vi "正式LABVIEW_11_16_1.vi"() -> ()   [LabVIEW 2019]
uses:
  <vilib>/Instr/_visa.llb/VISA Configure Serial Port (Instr).vi
panel:
  out "?":picture
  out "?":picture
  in  "防撞":bool
  out "右前":dbl
  out "左前":dbl
  out "オ":dbl
  out "右":dbl
  in  "更新影片&影片重播":bool
  in  "選擇導覽目標":path
  in  "導覽影片":refnum<k7>(container)
  out "濕度值":string
  in  "輸入阜來源":refnum<visa-resource-name>
  in  "指紋辨識成功影片":refnum<k7>(container)
  in  "指紋辨識檔案":path
  out "溫度值":string
  out "濕度條":dbl(slide) scale=0.0..100.0
  out "溫度條":dbl(slide) scale=0.0..50.0
  out "右後":dbl
  out "左後":dbl
  in  "倒車雷達":bool
  in  "溫度濕度開關":bool
  in  "程式關閉":bool
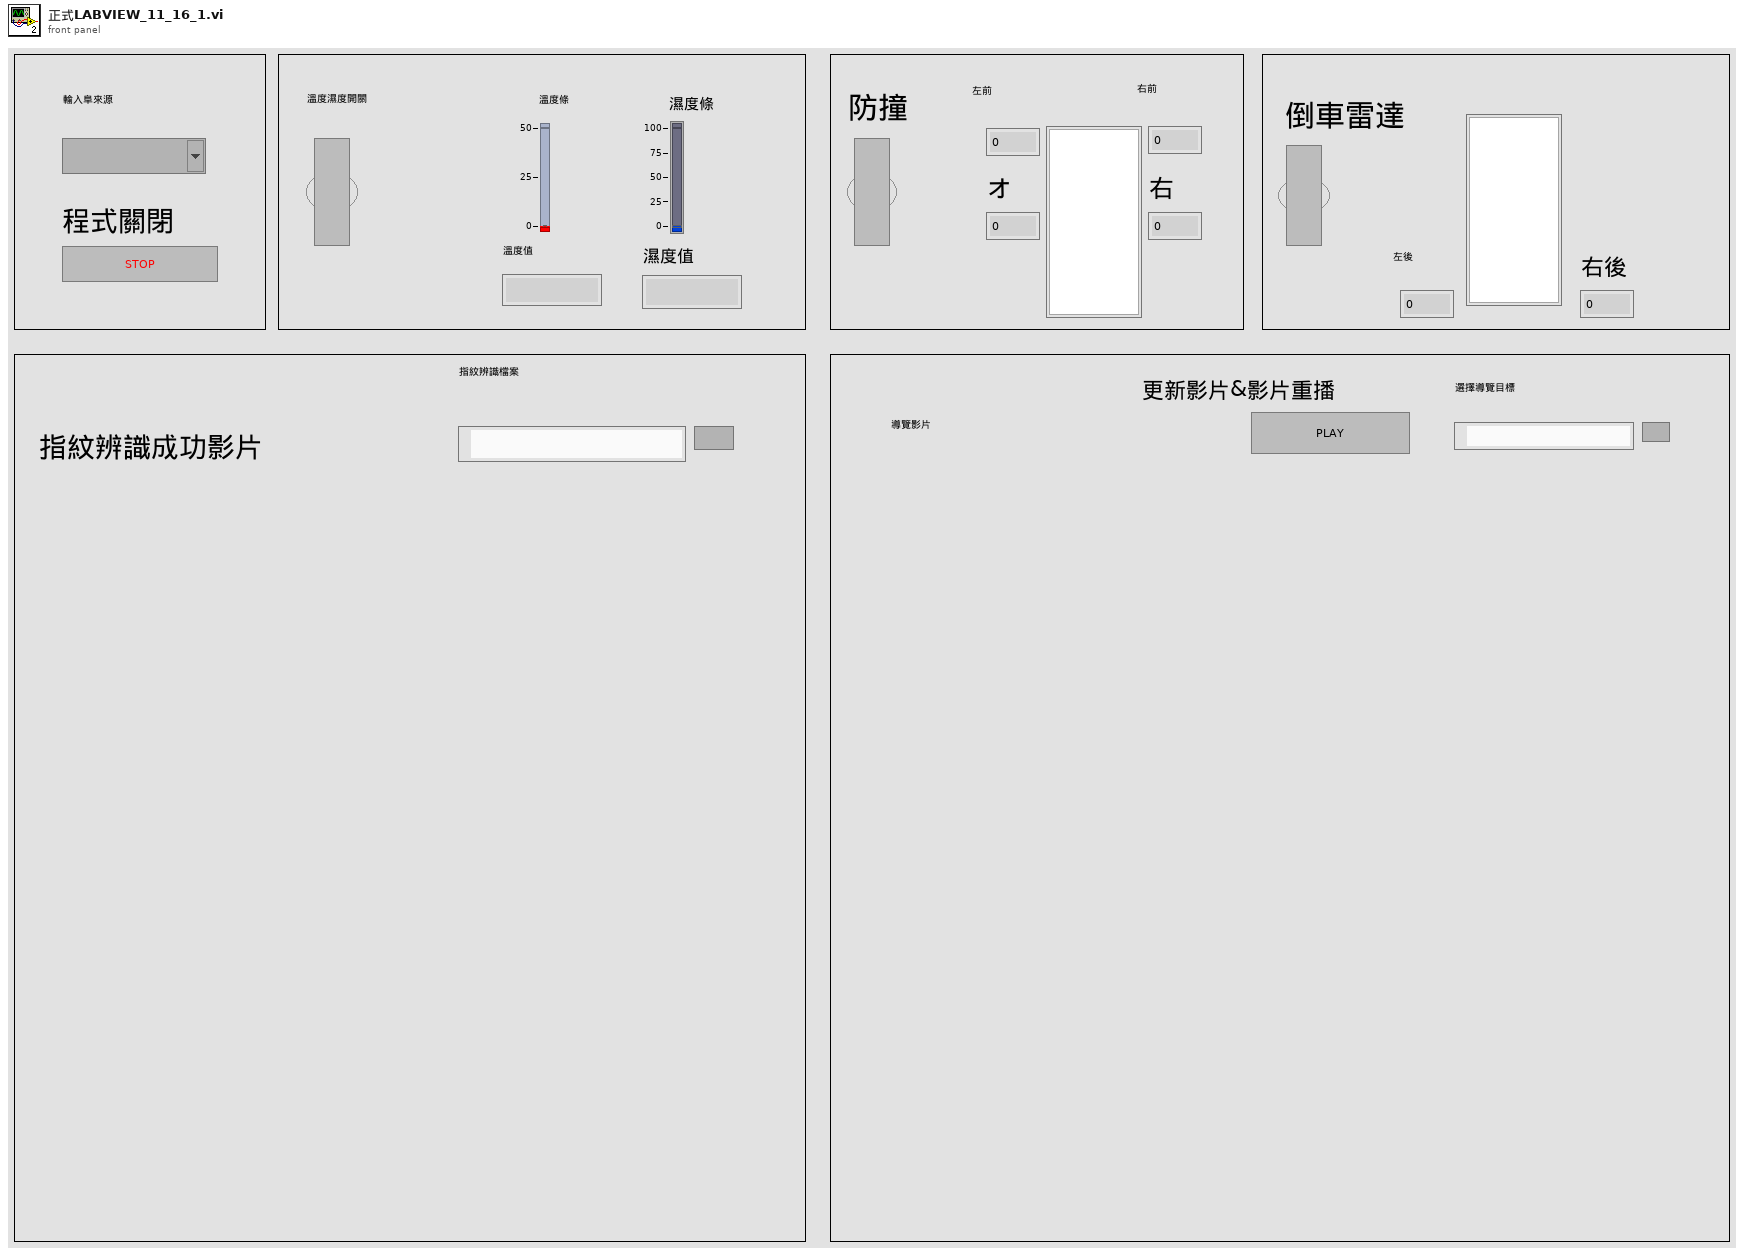
[diagram p1: front panel]
types:
  T1 = typedef "imagedata.ctl" = cluster{"image type":i32, "image depth":i32, "image":u8[], "mask":u8[], "colors":u32[], "Rectangle":cluster{"left":i16, "top":i16, "right":i16, "bottom":i16}}
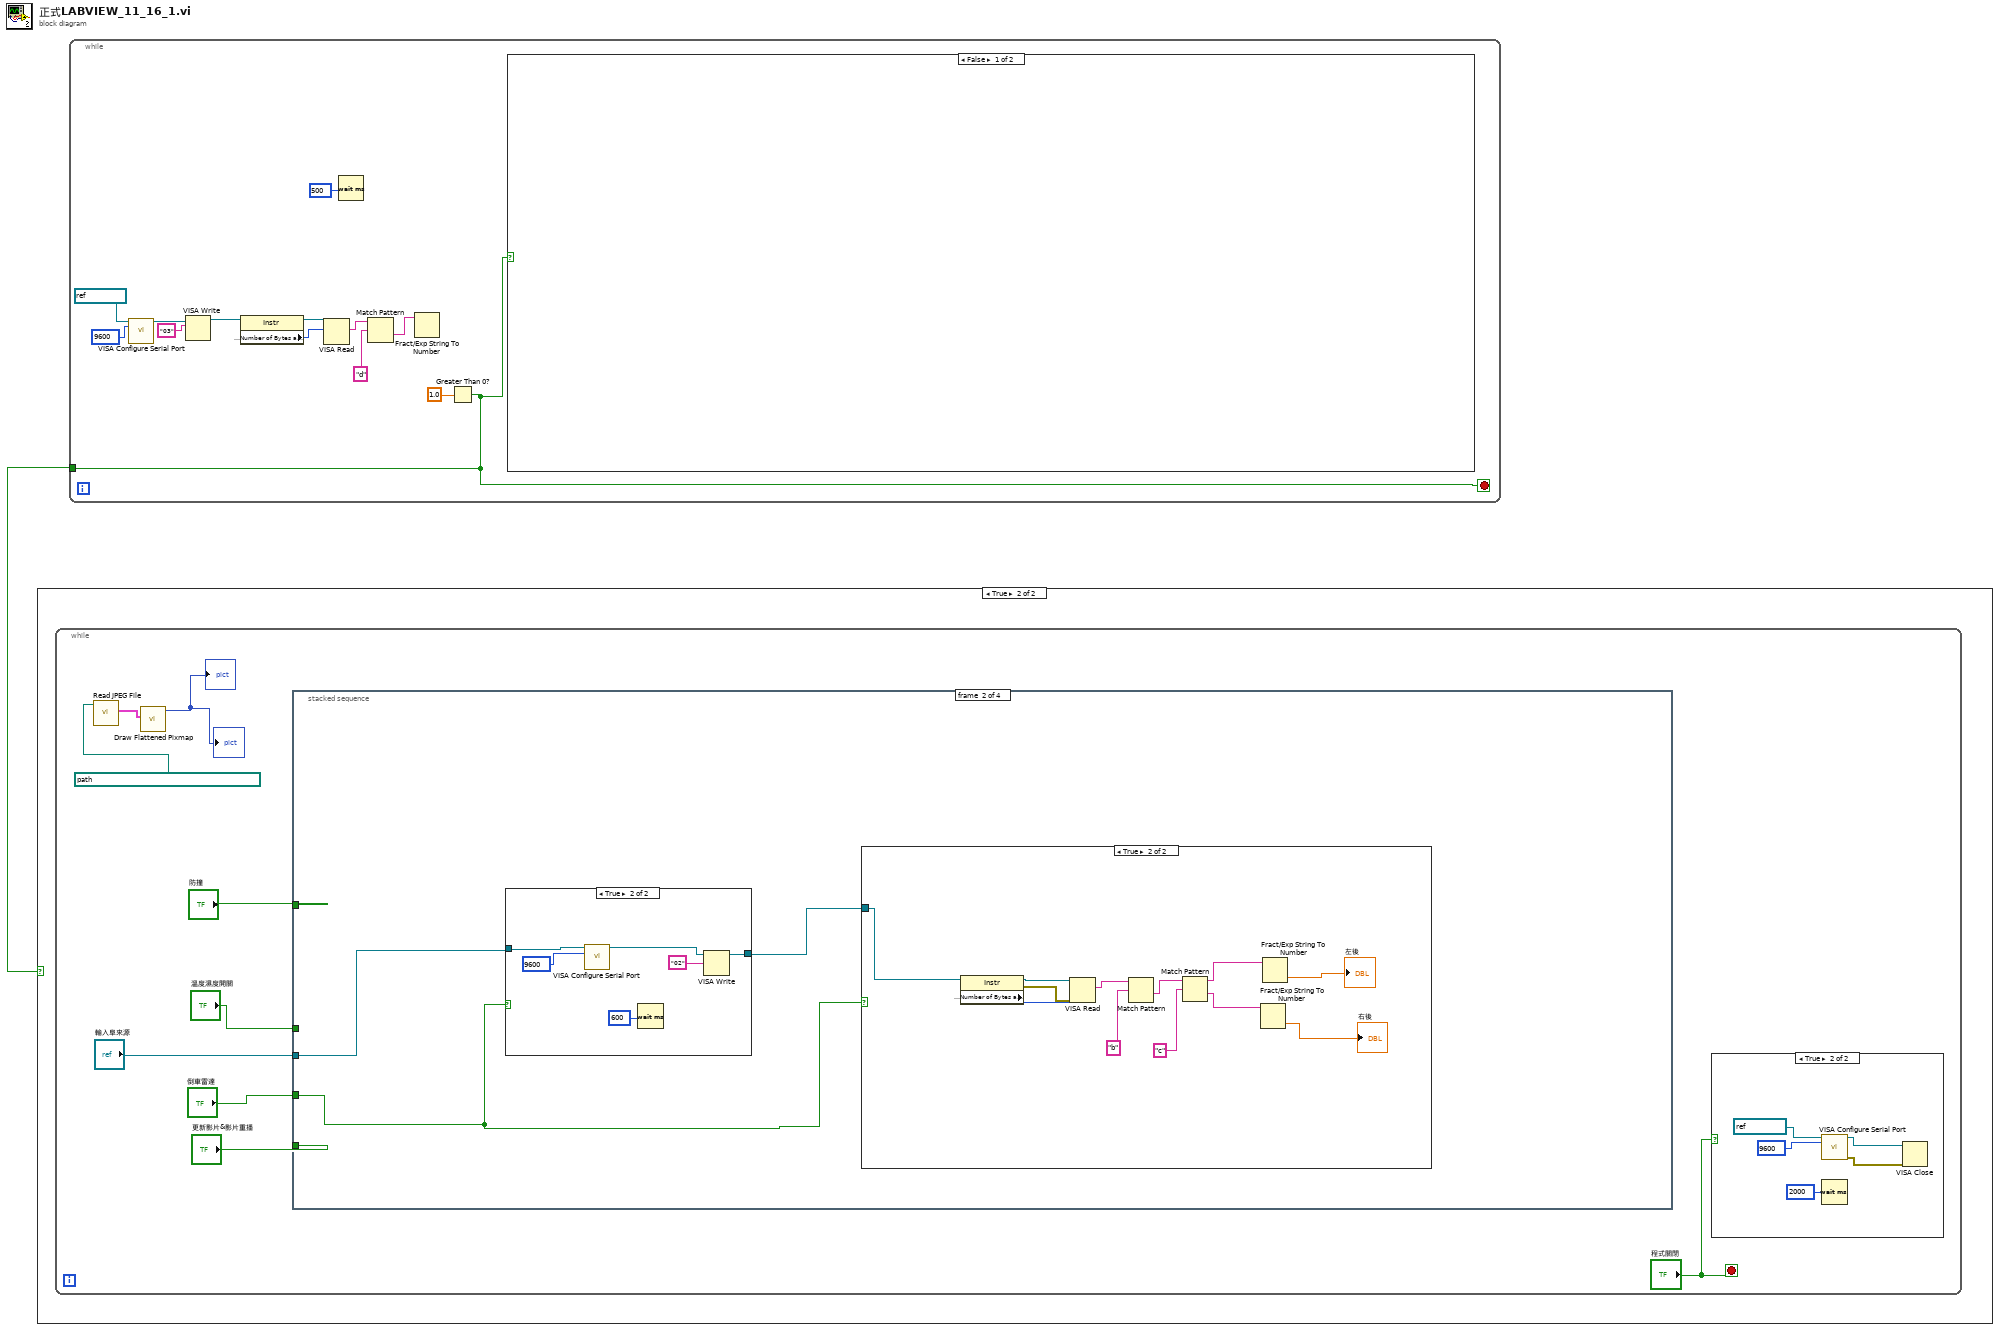
[diagram p0: block diagram]
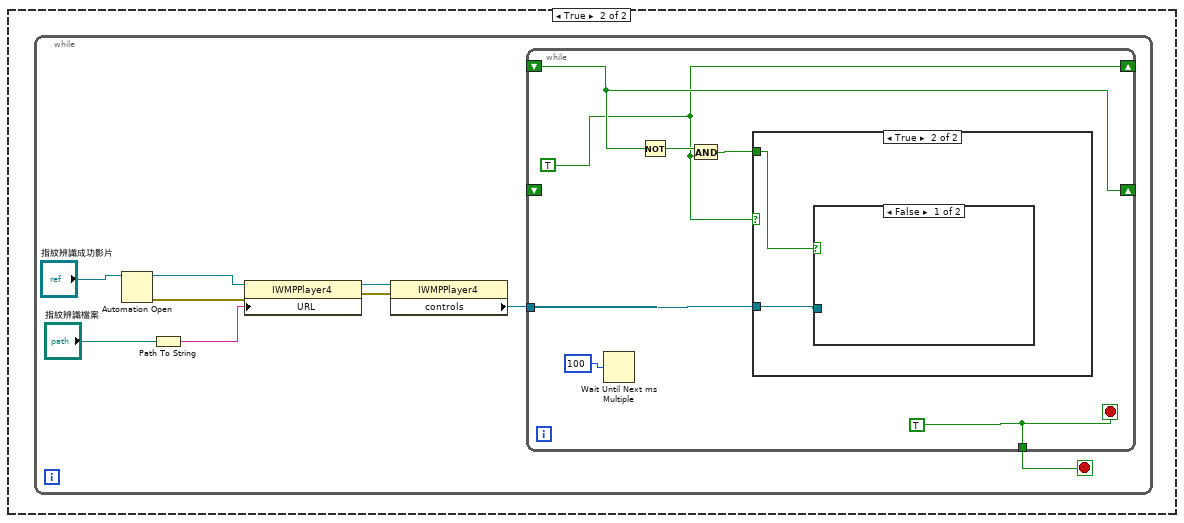
[diagram p2: hidden frame]
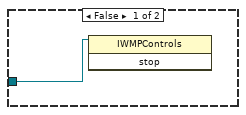
[diagram p3: hidden frame]
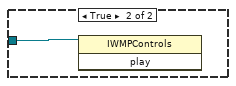
[diagram p4: hidden frame]
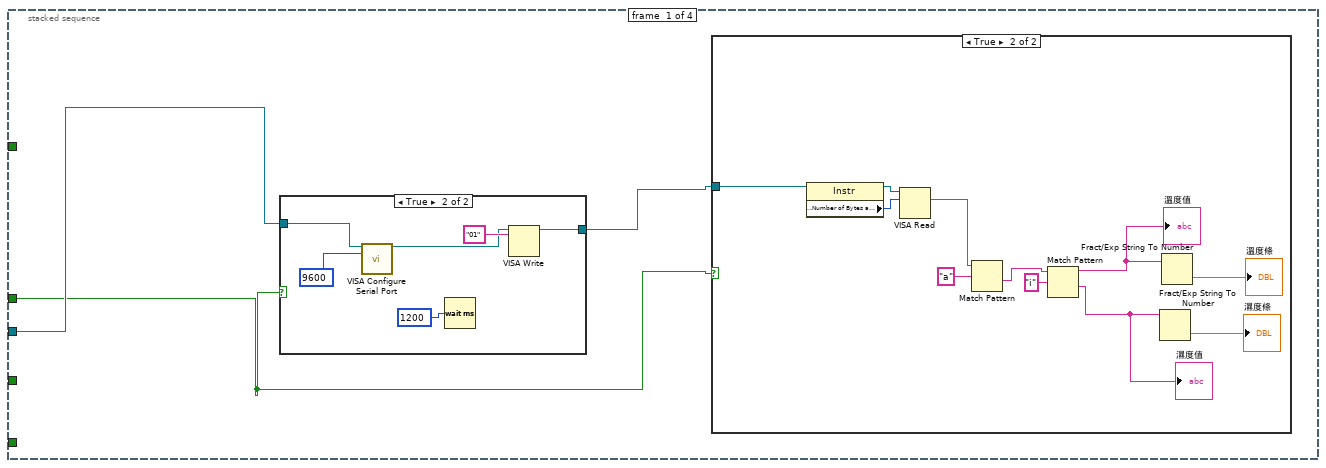
[diagram p7: hidden frame]
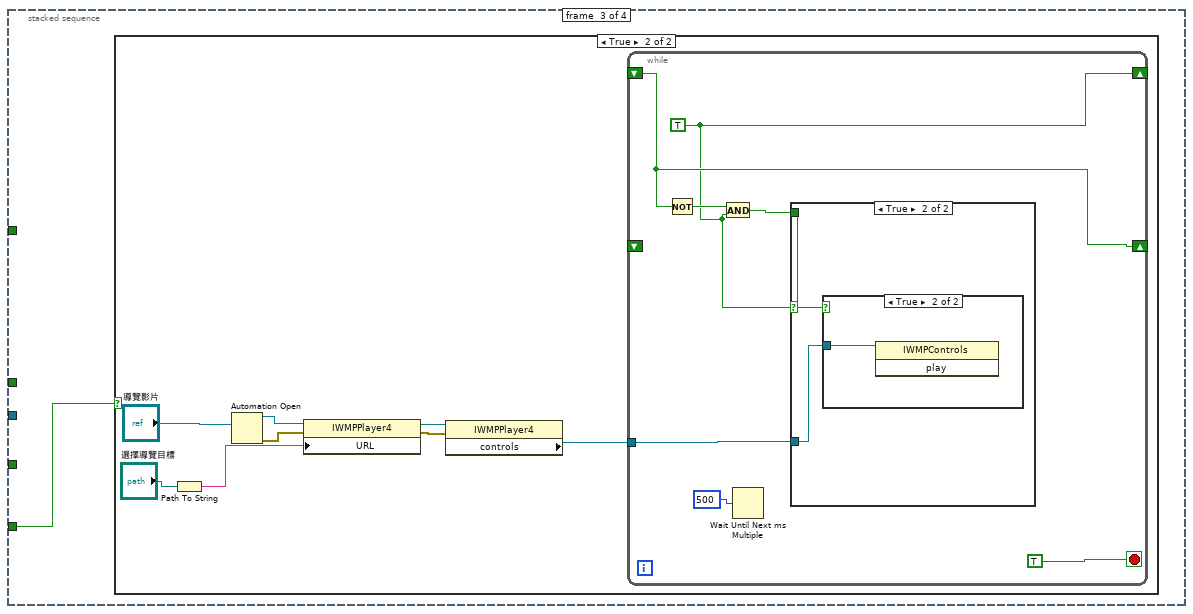
[diagram p12: hidden frame]
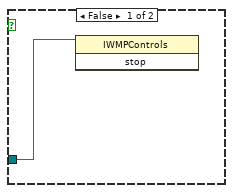
[diagram p14: hidden frame]
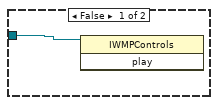
[diagram p15: hidden frame]
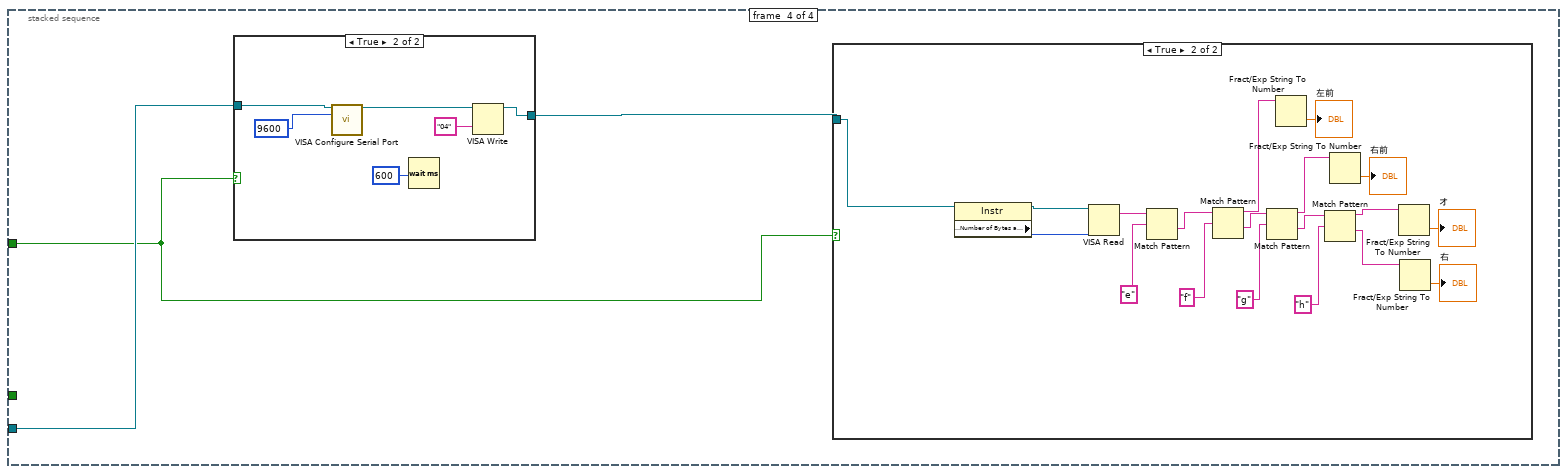
[diagram p16: hidden frame]
diagram:
  n1 = while {
    tunnel: [w2] -> w1
    stop <- w2 stop-if-true
    n2 = call-poly "VISA Configure Serial Port"("VISA resource name"=refnum<visa-resource-name> "COM6", "baud rate (9600)"=u32 9600) -> ("VISA resource name out"=w7:refnum<visa-resource-name>)  [unwired: 12 in, 1 out]
    n3 = VISA Write(VISA resource name=w7, write buffer="03") -> (VISA resource name out=w5:refnum<visa-resource-name>)  [unwired: 1 in, 2 out]
    n4 = property class="Instr"(reference=w5) -> (reference out=w13:refnum<visa-resource-name>, "Serial Settings:Number of Bytes at Serial Port"=w12:u32)  [unwired: 1 in, 1 out]
    n5 = VISA Read(VISA resource name=w13, byte count=w12) -> (read buffer=w11:string)  [unwired: 1 in, 3 out]
    n6 = Wait (ms)(milliseconds to wait=u32 500) -> ()  [unwired: 1 out]
    n7 = Match Pattern(string=w11, regular expression="d") -> (after substring=w10:string)  [unwired: 1 in, 3 out]
    n8 = Fract/Exp String To Number(string=w10) -> ()  [unwired: 3 in, 2 out]
    n9 = Greater Than 0?(x=1.0) -> (x > 0?=w2:bool)
    n10 = case shown="False" w2 {
      frame False {
      }
      frame True {
        n11 = while {
          stop <- w16 stop-if-true
          n12 = Automation Open(Automation Refnum="指紋辨識成功影片") -> (Automation Refnum=w18:refnum<k7>, error out=w20:errorcluster)  [unwired: 3 in]
          n13 = Path To String(path="指紋辨識檔案") -> (string=w22:string)
          n14 = property class="IWMPPlayer4"(reference=w18, error in=w20, "URL"=w22) -> (reference out=w19:refnum<k7>, error out=w21:errorcluster)
          n15 = property class="IWMPPlayer4"(reference=w19, error in=w21) -> ("controls"=w17:refnum<k7>)  [unwired: 2 out]
          n16 = while {
            tunnel: w17 -> [w30]
            shift-right: [w27] -> _
            shift-left: _ -> [_]
            shift-right: [w25] -> _
            shift-left: _ -> [w27]
            tunnel: [w24] -> w16
            stop <- w24 stop-if-true
            w24 = TRUE
            w25 = TRUE
            n17 = Wait Until Next ms Multiple(millisecond multiple=u32 100 ("millisecond timer value")) -> ()  [unwired: 1 out]
            n18 = Not(x=w27) -> (.not. x?=w29:bool)
            n19 = And(x=w29, y=w25) -> (x .and. y?=w28:bool)
            n20 = case shown="True" w25 {
              tunnel: w30 -> [w31 w33]
              tunnel: w28 -> [_ w32]
              frame False {
                n21 = invoke class="IWMPControls" method="stop"(reference=w31) -> ()  [unwired: 2 in, 3 out]
              }
              frame True {
                n22 = case shown="False" w32 {
                  tunnel: w33 -> [_ w34]
                  frame False {
                  }
                  frame True {
                    n23 = invoke class="IWMPControls" method="play"(reference=w34) -> ()  [unwired: 2 in, 3 out]
                  }
                }
              }
            }
          }
        }
      }
    }
  }
  n24 = case shown="True" w1 {
    frame False {
    }
    frame True {
      n25 = while {
        stop <- "程式關閉" stop-if-true
        n26 = call <vilib>:"Read JPEG File.vi"("path to JPEG file"=path "D:/AA708/06371025/模擬車府試圖.jpg") -> ("image data"=w40:T1)  [unwired: 8 in, 2 out]
        n27 = call <vilib>:"Draw Flattened Pixmap.vi"("image data"=w40) -> ("new picture"=→"?" →"?":picture)  [unwired: 8 in]
        n28 = stacked-sequence {
          tunnel: "倒車雷達" -> [_ w70 _ _]
          tunnel: "輸入阜來源" -> [w51 w72 _ w115]
          tunnel: "更新影片&影片重播" -> [_ _ w92 _]
          tunnel: "防撞" -> [_ _ _ w113]
          tunnel: "溫度濕度開關" -> [w49 _ _ _]
          frame #0 {
            n29 = case shown="True" w49 {
              tunnel: w51 -> [w52 w55]
              tunnel: [w52 w54] -> w50
              frame False {
              }
              frame True {
                n30 = call-poly "VISA Configure Serial Port"("VISA resource name"=w55, "baud rate (9600)"=u32 9600) -> ("VISA resource name out"=w56:refnum<visa-resource-name>)  [unwired: 12 in, 1 out]
                n31 = Wait (ms)(milliseconds to wait=u32 1200) -> ()  [unwired: 1 out]
                n32 = VISA Write(VISA resource name=w56, write buffer="01") -> (VISA resource name out=w54:refnum<visa-resource-name>)  [unwired: 1 in, 2 out]
              }
            }
            n33 = case shown="True" w49 {
              tunnel: w50 -> [_ w63]
              frame False {
              }
              frame True {
                n34 = property class="Instr"(reference=w63) -> (reference out=w65:refnum<visa-resource-name>, "Serial Settings:Number of Bytes at Serial Port"=w64:u32)  [unwired: 1 in, 1 out]
                n35 = VISA Read(VISA resource name=w65, byte count=w64) -> (read buffer=w66:string)  [unwired: 1 in, 3 out]
                n36 = Match Pattern(string=w66, regular expression="a") -> (after substring=w61:string)  [unwired: 1 in, 3 out]
                n37 = Match Pattern(string=w61, regular expression="i") -> (before substring=w60:string, after substring=w59:string)  [unwired: 1 in, 2 out]
                "溫度值" <- w60
                "濕度值" <- w59
                n38 = Fract/Exp String To Number(string=w59) -> (number=→"濕度條":dbl)  [unwired: 3 in, 1 out]
                n39 = Fract/Exp String To Number(string=w60) -> (number=→"溫度條":dbl)  [unwired: 3 in, 1 out]
              }
            }
          }
          frame #1 {
            n40 = case shown="True" w70 {
              tunnel: [w73 w78] -> w71
              tunnel: w72 -> [w73 w77]
              frame False {
              }
              frame True {
                n41 = call-poly "VISA Configure Serial Port"("VISA resource name"=w77, "baud rate (9600)"=u32 9600) -> ("VISA resource name out"=w75:refnum<visa-resource-name>)  [unwired: 12 in, 1 out]
                n42 = Wait (ms)(milliseconds to wait=u32 600) -> ()  [unwired: 1 out]
                n43 = VISA Write(VISA resource name=w75, write buffer="02") -> (VISA resource name out=w78:refnum<visa-resource-name>)  [unwired: 1 in, 2 out]
              }
            }
            n44 = case shown="True" w70 {
              tunnel: w71 -> [_ w86]
              frame False {
              }
              frame True {
                n45 = property class="Instr"(reference=w86) -> (reference out=w91:refnum<visa-resource-name>, error out=w90:errorcluster, "Serial Settings:Number of Bytes at Serial Port"=w89:u32)  [unwired: 1 in]
                n46 = VISA Read(VISA resource name=w91, byte count=w89, error in (no error)=w90) -> (read buffer=w87:string)  [unwired: 3 out]
                n47 = Match Pattern(string=w87, regular expression="b") -> (after substring=w85:string)  [unwired: 1 in, 3 out]
                n48 = Match Pattern(string=w85, regular expression="c") -> (before substring=w83:string, after substring=w82:string)  [unwired: 1 in, 2 out]
                n49 = Fract/Exp String To Number(string=w82) -> (number=→"右後":dbl)  [unwired: 3 in, 1 out]
                n50 = Fract/Exp String To Number(string=w83) -> (number=→"左後":dbl)  [unwired: 3 in, 1 out]
              }
            }
          }
          frame #2 {
            n51 = case shown="True" w92 {
              frame False {
              }
              frame True {
                n52 = Path To String(path="選擇導覽目標") -> (string=w99:string)
                n53 = Automation Open(Automation Refnum="導覽影片") -> (Automation Refnum=w95:refnum<k7>, error out=w97:errorcluster)  [unwired: 3 in]
                n54 = property class="IWMPPlayer4"(reference=w95, error in=w97, "URL"=w99) -> (reference out=w96:refnum<k7>, error out=w98:errorcluster)
                n55 = property class="IWMPPlayer4"(reference=w96, error in=w98) -> ("controls"=w93:refnum<k7>)  [unwired: 2 out]
                n56 = while {
                  tunnel: w93 -> [w107]
                  shift-right: [w103] -> _
                  shift-left: _ -> [_]
                  shift-right: [w102] -> _
                  shift-left: _ -> [w103]
                  stop <- TRUE stop-if-true
                  w102 = TRUE
                  n57 = Not(x=w103) -> (.not. x?=w106:bool)
                  n58 = And(x=w106, y=w102) -> (x .and. y?=w105:bool)
                  n59 = Wait Until Next ms Multiple(millisecond multiple=u32 500 ("millisecond timer value")) -> ()  [unwired: 1 out]
                  n60 = case shown="True" w102 {
                    tunnel: w107 -> [w108 w110]
                    tunnel: w105 -> [_ w109]
                    frame False {
                      n61 = invoke class="IWMPControls" method="stop"(reference=w108) -> ()  [unwired: 2 in, 3 out]
                    }
                    frame True {
                      n62 = case shown="True" w109 {
                        tunnel: w110 -> [w111 w112]
                        frame False {
                          n63 = invoke class="IWMPControls" method="play"(reference=w111) -> ()  [unwired: 2 in, 3 out]
                        }
                        frame True {
                          n64 = invoke class="IWMPControls" method="play"(reference=w112) -> ()  [unwired: 2 in, 3 out]
                        }
                      }
                    }
                  }
                }
              }
            }
          }
          frame #3 {
            n65 = case shown="True" w113 {
              tunnel: [w116 w121] -> w114
              tunnel: w115 -> [w116 w118]
              frame False {
              }
              frame True {
                n66 = call-poly "VISA Configure Serial Port"("VISA resource name"=w118, "baud rate (9600)"=u32 9600) -> ("VISA resource name out"=w119:refnum<visa-resource-name>)  [unwired: 12 in, 1 out]
                n67 = Wait (ms)(milliseconds to wait=u32 600) -> ()  [unwired: 1 out]
                n68 = VISA Write(VISA resource name=w119, write buffer="04") -> (VISA resource name out=w121:refnum<visa-resource-name>)  [unwired: 1 in, 2 out]
              }
            }
            n69 = case shown="True" w113 {
              tunnel: w114 -> [_ w136]
              frame False {
              }
              frame True {
                n70 = property class="Instr"(reference=w136) -> (reference out=w141:refnum<visa-resource-name>, "Serial Settings:Number of Bytes at Serial Port"=w140:u32)  [unwired: 1 in, 1 out]
                n71 = VISA Read(VISA resource name=w141, byte count=w140) -> (read buffer=w123:string)  [unwired: 1 in, 3 out]
                n72 = Match Pattern(string=w123, regular expression="e") -> (after substring=w135:string)  [unwired: 1 in, 3 out]
                n73 = Match Pattern(string=w135, regular expression="f") -> (before substring=w130:string, after substring=w131:string)  [unwired: 1 in, 2 out]
                n74 = Match Pattern(string=w131, regular expression="g") -> (before substring=w128:string, after substring=w129:string)  [unwired: 1 in, 2 out]
                n75 = Fract/Exp String To Number(string=w130) -> (number=→"左前":dbl)  [unwired: 3 in, 1 out]
                n76 = Match Pattern(string=w129, regular expression="h") -> (before substring=w126:string, after substring=w124:string)  [unwired: 1 in, 2 out]
                n77 = Fract/Exp String To Number(string=w128) -> (number=→"右前":dbl)  [unwired: 3 in, 1 out]
                n78 = Fract/Exp String To Number(string=w126) -> (number=→"オ":dbl)  [unwired: 3 in, 1 out]
                n79 = Fract/Exp String To Number(string=w124) -> (number=→"右":dbl)  [unwired: 3 in, 1 out]
              }
            }
          }
        }
        n80 = case shown="True" "程式關閉" {
          frame False {
          }
          frame True {
            n81 = call-poly "VISA Configure Serial Port"("VISA resource name"=refnum<visa-resource-name> "COM6", "baud rate (9600)"=u32 9600) -> ("VISA resource name out"=w45:refnum<visa-resource-name>, "error out"=w44:errorcluster)  [unwired: 12 in]
            n82 = Wait (ms)(milliseconds to wait=u32 2000) -> ()  [unwired: 1 out]
            n83 = VISA Close(VISA resource name=w45, error in (no error)=w44) -> ()  [unwired: 1 out]
          }
        }
      }
    }
  }
